vi "OnlyPhidget.vi"() -> ()   [LabVIEW 2013]
panel:
  out "error out":errorcluster
  in  "Stop":bool
  in  "Enabled":bool
  in  "Voltage":dbl(slide) scale=-10.0..10.0
  in  "Channel #:":u16(ring) items=["0", "1", "2", "3"]
  out "Output":T1(array[cluster])
  out "#Channels:":i32
  out "Attached?":bool
  out "Serial Number":i32
  # "This example is designed for 1002"
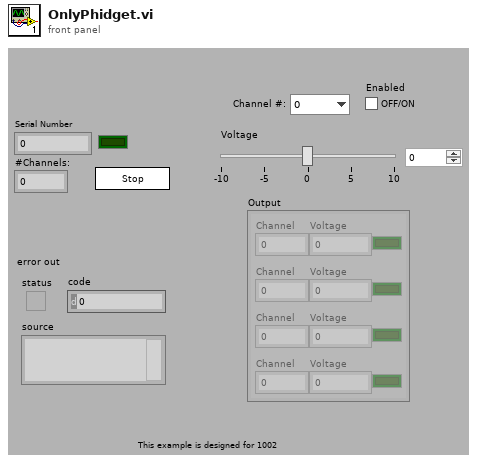
[diagram p1: front panel]
types:
  T1 = cluster{"Channel":i32, "Voltage":dbl, "Enabled?":bool}[]
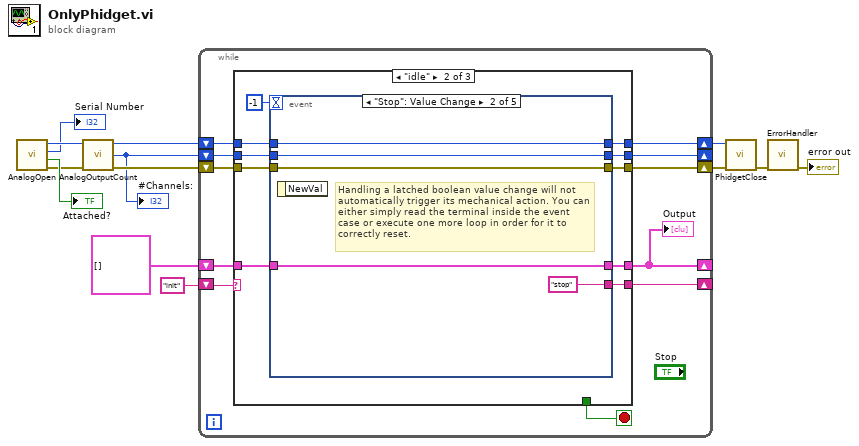
[diagram p0: block diagram]
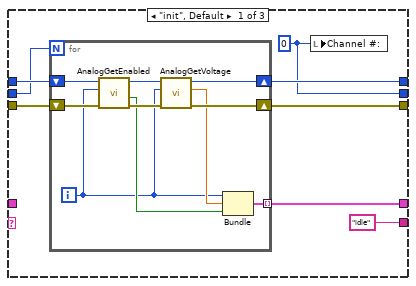
[diagram p2: hidden frame]
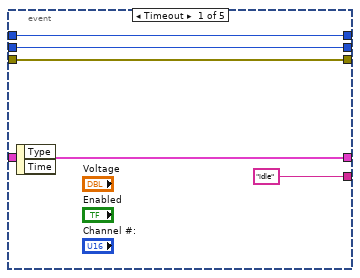
[diagram p3: hidden frame]
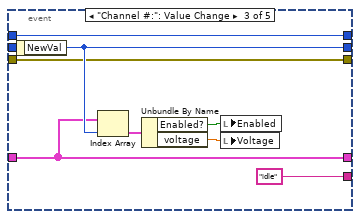
[diagram p4: hidden frame]
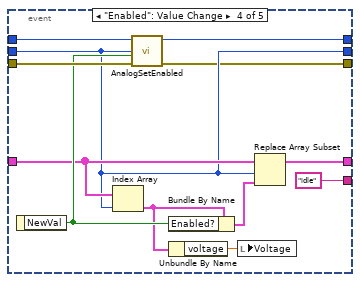
[diagram p5: hidden frame]
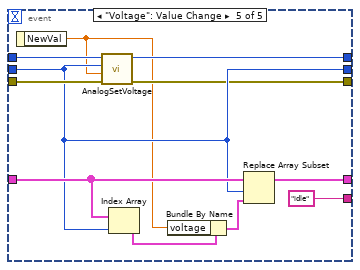
[diagram p6: hidden frame]
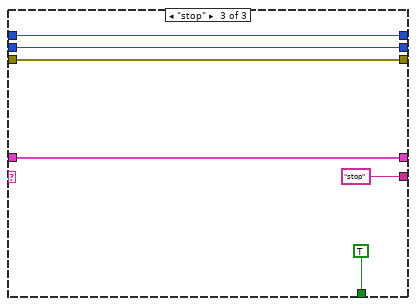
[diagram p7: hidden frame]
diagram:
  n1 = call "AnalogOpen.vi"() -> ("error out"=w5:errorcluster, "Attached?"=→"Attached?":bool, "Serial Number Return"=→"Serial Number":i32, "Device Out"=w13:i32)  [unwired: 8 in]
  n2 = call "AnalogOutputCount.vi"("error in (no error)"=w5, "Device In"=w13) -> ("error out"=w9:errorcluster, "Count"=w8:i32, "Device Out"=w10:i32)  [unwired: 7 in]
  "#Channels:" <- w8
  n3 = while {
    shift-right: [w19] -> w3
    shift-left: w9 -> [w23]
    shift-right: [w22] -> w4
    shift-left: w10 -> [w24]
    shift-right: [w16] -> _
    shift-left: "init" -> [w20]
    shift-right: [w18] -> _
    shift-left: cluster{i32, "voltage":dbl, "Enabled?":bool}[] [] -> [w15]
    shift-right: [w17] -> _
    shift-left: w8 -> [w21]
    stop <- w14 stop-if-true
    n4 = case shown="\"idle\"" w20 {
      tunnel: w24 -> [w32 w49 w98]
      tunnel: w23 -> [w31 w47 w94]
      tunnel: [w30 w50 w96] -> w18
      tunnel: [w29 w48 w98] -> w22
      tunnel: w21 -> [w28 w45 w97]
      tunnel: [w27 w46 w94] -> w19
      tunnel: [w26 w51 w97] -> w17
      tunnel: ["idle" w44 "stop"] -> w16
      tunnel: w15 -> [_ w52 w96]
      tunnel: [_ _ TRUE ("Stop")] -> w14
      frame "init", Default {
        w26 = 0
        n5 = for {
          N: w28 -> [_]
          shift-right: [w38] -> w27
          shift-left: w31 -> [w39]
          shift-right: [w37] -> w29
          shift-left: w32 -> [w42]
          tunnel: [w33] -> w30 mode=indexing
          i -> [w34]
          n6 = call "AnalogGetEnabled.vi"("error in (no error)"=w39, "index"=w34, "Device In"=w42) -> ("error out"=w40:errorcluster, "Enabled?"=w35:bool, "Device Out"=w41:i32)  [unwired: 4 in, 1 out]
          n7 = call "AnalogGetVoltage.vi"("error in (no error)"=w40, "index"=w34, "Device In"=w41) -> ("error out"=w38:errorcluster, "voltage"=w36:dbl, "Device Out"=w37:i32)  [unwired: 5 in]
          n8 = Bundle(w34, "voltage"=w36, "Enabled?"=w35) -> (w33:cluster{i32, "voltage":dbl, "Enabled?":bool})  [unwired: 1 in]
        }
        n9 = local write "Channel #:"(w26) -> ()
      }
      frame "idle" {
        n10 = event shown="[1] \"Stop\": Value Change" {
          selector: _ -> [_ _ _ _ _]
          dyn-events: _ -> [_ _ _ _ _]
          timeout: -1 -> [_ _ _ _ _]
          tunnel: w52 -> [w53 w62 w66 w80 w89]
          tunnel: [w56 w59 w70 w75 w86] -> w51
          tunnel: [w53 w62 w66 w78 w87] -> w50
          tunnel: w49 -> [w57 w61 w64 w76 w92]
          tunnel: [w57 w61 w64 w74 w84] -> w48
          tunnel: w47 -> [w55 w60 w63 w82 w93]
          tunnel: [w55 w60 w63 w73 w85] -> w46
          tunnel: w45 -> [w56 w59 _ w75 w86]
          tunnel: ["idle" "stop" "idle" "idle" "idle"] -> w44
          event Timeout {
            n11 = event-data() -> ()  [unwired: 1 in, 2 out]
          }
          event "Stop": Value Change {
            # "Handling a latched boolean value change will not automatically trigger its mechanical action. You can either simply read the terminal inside the event case or execute one more loop in order for it to correctly reset."
            n12 = event-data() -> ()  [unwired: 1 in, 1 out]
          }
          event "Channel #:": Value Change {
            n13 = event-data() -> ("NewVal"=w70:u16)  [unwired: 1 in]
            n14 = Index Array(array=w66, index=w70) -> (element=w69:cluster{i32, "voltage":dbl, "Enabled?":bool})
            n15 = Unbundle By Name(w69) -> ("Enabled?"=w68:bool, "voltage"=w67:dbl)
            n16 = local write "Enabled"(w68) -> ()
            n17 = local write "Voltage"(w67) -> ()
          }
          event "Enabled": Value Change {
            n18 = event-data() -> ("NewVal"=w81:bool)  [unwired: 1 in]
            n19 = Index Array(array=w80, index=w75) -> (element=w72:cluster{i32, "voltage":dbl, "Enabled?":bool})
            n20 = call "AnalogSetEnabled.vi"("error in (no error)"=w82, "SetEnabled"=w81, "index"=w75, "Device In"=w76) -> ("error out"=w73:errorcluster, "Device Out"=w74:i32)  [unwired: 5 in]
            n21 = Bundle By Name(cluster=w72, "Enabled?"=w81) -> (w79:cluster{i32, "voltage":dbl, "Enabled?":bool})
            n22 = Unbundle By Name(w72) -> ("voltage"=w71:dbl)
            n23 = local write "Voltage"(w71) -> ()
            n24 = Replace Array Subset(array=w80, new element=w79, index=w75) -> (w78:cluster{i32, "voltage":dbl, "Enabled?":bool}[])
          }
          event "Voltage": Value Change {
            n25 = event-data() -> ("NewVal"=w83:dbl)  [unwired: 1 in]
            n26 = call "AnalogSetVoltage.vi"("error in (no error)"=w93, "voltage"=w83, "index"=w86, "Device In"=w92) -> ("error out"=w85:errorcluster, "Device Out"=w84:i32)  [unwired: 5 in]
            n27 = Index Array(array=w89, index=w86) -> (element=w90:cluster{i32, "voltage":dbl, "Enabled?":bool})
            n28 = Bundle By Name(cluster=w90, "voltage"=w83) -> (w88:cluster{i32, "voltage":dbl, "Enabled?":bool})
            n29 = Replace Array Subset(array=w89, new element=w88, index=w86) -> (w87:cluster{i32, "voltage":dbl, "Enabled?":bool}[])
          }
        }
      }
      frame "stop" {
      }
    }
    "Output" <- w18
  }
  n30 = call "PhidgetClose.vi"("error in"=w3, "Device In"=w4) -> ("error out"=w2:errorcluster)  [unwired: 9 in]
  n31 = call "ErrorHandler.vi"("error in"=w2) -> ("error out"=→"error out":errorcluster)  [unwired: 9 in, 1 out]
